vi "参数初始化.vi"(8 "error in (no error)":errorcluster caption="错误输入（无错误）") -> (0 "error out":errorcluster caption="错误输出")   [LabVIEW 2016, in "main.lvlib"]
uses:
  main.lvlib
  DST800/DST800.lvlib
  EXO2/EXO2.lvlib
  bbe/bbe.lvlib
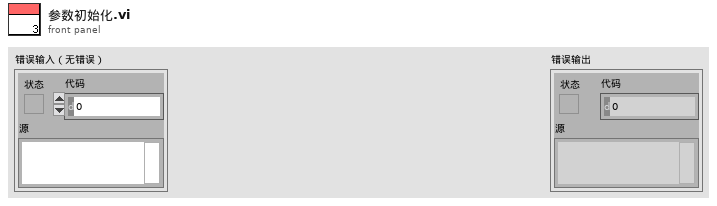
[diagram p1: front panel]
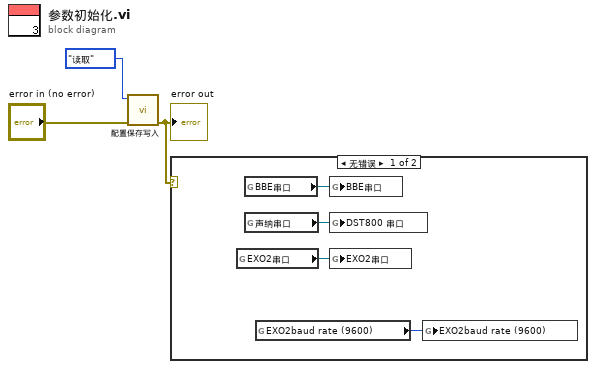
[diagram p0: block diagram]
diagram:
  n1 = call "配置保存写入.vi"("error in (no error)"="error in (no error)", "配置"=enum16{"读取", "写入"}."读取") -> ("error out"=w2:errorcluster)  [unwired: 9 in]
  "error out" <- w2
  n2 = case shown="无错误" w2 {
    frame No Error {
      n3 = global read "全局断电保存变量.vi" "EXO2串口"() -> (w5:refnum<visa-resource-name>)
      n4 = global read "全局断电保存变量.vi" "BBE串口"() -> (w4:refnum<visa-resource-name>)
      n5 = global read "全局断电保存变量.vi" "声纳串口"() -> (w7:refnum<visa-resource-name>)
      n6 = global read "全局断电保存变量.vi" "EXO2baud rate (9600)"() -> (w6:u32)
      n7 = global write "过程变量.vi" "BBE串口"(w4) -> ()
      n8 = global write "DST800全局变量.vi" "DST800 串口"(w7) -> ()
      n9 = global write "EXO2全局变量.vi" "EXO2串口"(w5) -> ()
      n10 = global write "EXO2全局变量.vi" "EXO2baud rate (9600)"(w6) -> ()
    }
    frame Error {
    }
  }
